vi "PythonNode_AddTwoIntegers.vi"() -> ()   [LabVIEW 2023]
doc: "This example demonstrates how to call a Python function and pass integers as arguments. It uses a python function to compute the sum of two integers."
uses:
  Program Files (x86)/National Instruments/LabVIEW 2023/examples/Connectivity/Python/support/PythonVersionsEnum.ctl
panel:
  out "error out":errorcluster
  out "a + b":i32
  in  "b":i32=1
  in  "a":i32=41
  in  "error in (no error)":errorcluster
  in  "python version":T1
  # "Overview: Demonstrates how to call a Python function and pass int32s as arguments.\nRequirements: Python 3.6, 3.7, 3.8, 3.9 or 3.10 with the same bitness as LabVIEW.\nInstructions:\n1. Set the Python version to the version of Python you want to execute code in.\n2. Run the VI. You should see the result of adding \"a\" and \"b\" in the indicator \"a + b\".\n3. See comments on the block diagram of this VI and in \"ExamplePythonModule.py\" for more information about how the call python node passes arguments and handles return values."
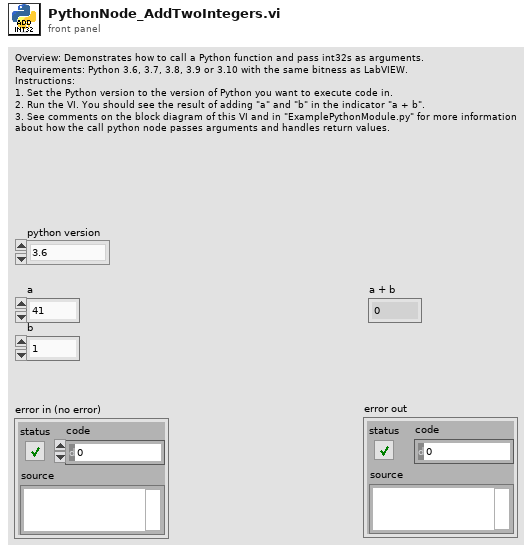
[diagram p1: front panel]
types:
  T1 = typedef "PythonVersionsEnum.ctl" = enum16{"3.6", "3.7", "3.8", "3.9", "3.10"}
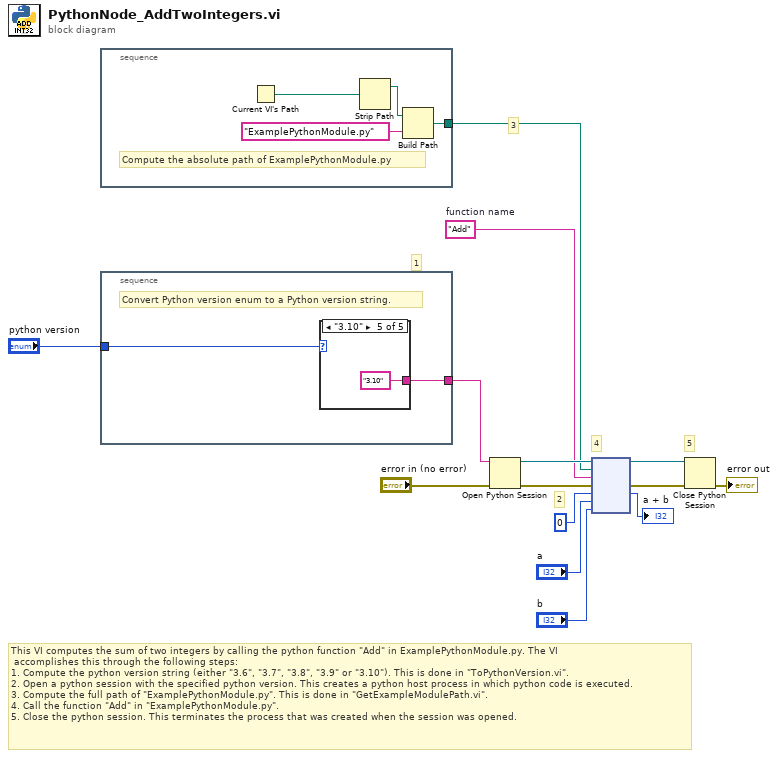
[diagram p0: block diagram]
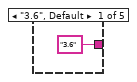
[diagram p2: hidden frame]
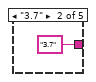
[diagram p3: hidden frame]
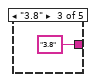
[diagram p4: hidden frame]
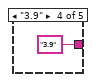
[diagram p5: hidden frame]
diagram:
  w8 = "Add"  # function name
  # "5"
  # "4"
  # "2"
  # "3"
  # "1"
  # "This VI computes the sum of two integers by calling the python function \"Add\" in ExamplePythonModule.py. The VI\n accomplishes this through the following steps:\n1. Compute the python version string (either \"3.6\", \"3.7\", \"3.8\", \"3.9\" or \"3.10\"). This is done in \"ToPythonVersion.vi\". \n2. Open a python session with the specified python version. This creates a python host process in which python code is executed.\n3. Compute the full path of \"ExamplePythonModule.py\". This is done in \"GetExampleModulePath.vi\".\n4. Call the function \"Add\" in \"ExamplePythonModule.py\".\n5. Close the python session. This terminates the process that was created when the session was opened."
  n1 = stacked-sequence {
    tunnel: [w18] -> w9
    frame #0 {
      # "Compute the absolute path of ExamplePythonModule.py"
      n2 = Current VI's Path() -> (path=w15:path)
      n3 = Strip Path(path=w15) -> (stripped path=w16:path)  [unwired: 1 out]
      n4 = Build Path(base path=w16, name or relative path="ExamplePythonModule.py") -> (appended path=w18:path)
    }
  }
  n5 = stacked-sequence {
    tunnel: [w20] -> w14
    tunnel: "python version" -> [w19]
    frame #0 {
      # "Convert Python version enum to a Python version string."
      n6 = case shown="\"3.10\"" w19 {
        tunnel: ["3.6" ("python version") "3.7" ("python version") "3.8" ("python version") "3.9" ("python version") "3.10" ("python version")] -> w20
        frame "3.6", Default {
        }
        frame "3.7" {
        }
        frame "3.8" {
        }
        frame "3.9" {
        }
        frame "3.10" {
        }
      }
    }
  }
  n7 = Open Python Session(python version=w14, 3:"error in (no error)") -> (session out=w11:refnum<k35>, error out=w10:errorcluster)  [unwired: 1 in]
  n8 = node(w11, w9, w8, w10, 0 ("a"), "a", "b") -> (w7:refnum<k35>, w6:errorcluster, →"a + b":i32)  [unwired: 2 in, 2 out]
  n9 = Close Python Session(session in=w7, error in=w6) -> (11:→"error out":errorcluster)
